vi "FileInformation.vi"(0 "File Path":path, 11 "error in (no error)":errorcluster) -> (4 "FileInfo":string[](array[string]), 15 "error out":errorcluster)   [LabVIEW 2021]
doc: "This VI gives the file information such as last modified, type and size."
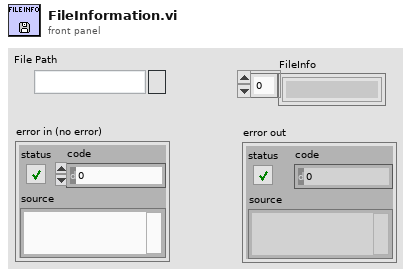
[diagram p1: front panel]
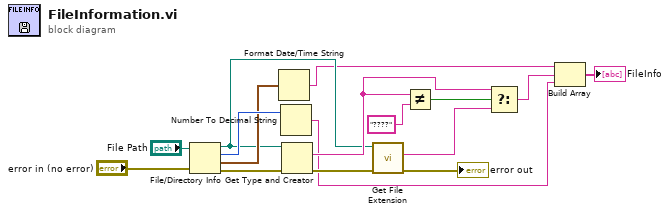
[diagram p0: block diagram]
diagram:
  n1 = File/Directory Info(path="File Path", error in="error in (no error)") -> (path out=w7:path, size=w14:i64, last mod=w13:timestamp, error out=w15:errorcluster)  [unwired: 3 out]
  n2 = Format Date/Time String(seconds (now)=w13) -> (date/time string=w5:string)  [unwired: 2 in]
  n3 = Number To Decimal String(number=w14) -> (decimal integer string=w3:string)  [unwired: 1 in]
  n4 = Get Type and Creator(4:w15, 7:w7) -> (0:w10:errorcluster, 2:w8:string)  [unwired: 2 out]
  n5 = call <vilib>:"Get File Extension.vi"("error in (no error)"=w10, "file"=w7) -> ("error out"=→"error out":errorcluster, "lowercase file extension"=w9:string)  [unwired: 5 in, 3 out]
  n6 = Not Equal?(x=w8, y="????") -> (x != y?=w11:bool)
  n7 = Select(t=w8, s=w11, f=w9) -> (s? t:f=w4:string)
  n8 = Build Array(w5, w4, w3) -> (→"FileInfo":string[])
